vi "Kinect Led Options.vi"(4 "Clear":bool, 6 "Rec":bool, 8 "States":T2, 9 "Bye active":bool, 10 "Bye inactive":bool) -> (0 "Led Option":T1)   [LabVIEW 2015]
uses:
  TypeDefs Host/States.ctl
  Kinect Support/Controls/Led Control.ctl
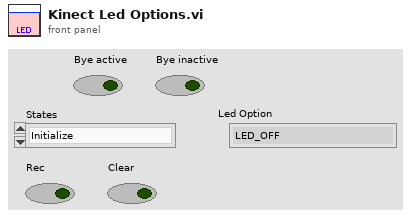
[diagram p1: front panel]
types:
  T1 = typedef "Led Control.ctl" = enum32{"LED_OFF", "LED_GREEN", "LED_RED", "LED_YELLOW", "LED_BLINK_GREEN", "LED_BLINK_GREEN2", "LED_BLINK_RED_YELLOW"}
  T2 = typedef "States.ctl" = enum16{"Initialize", "Calibrate", "Create", "Settings", "Shutdown"}
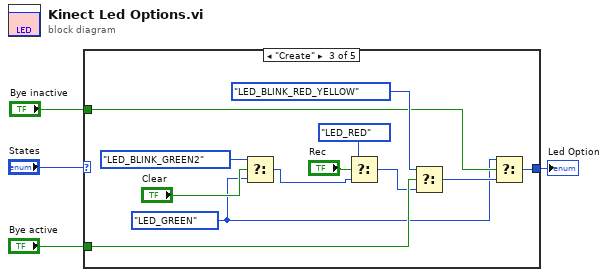
[diagram p0: block diagram]
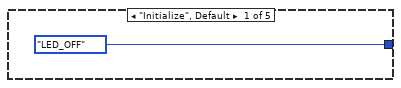
[diagram p2: hidden frame]
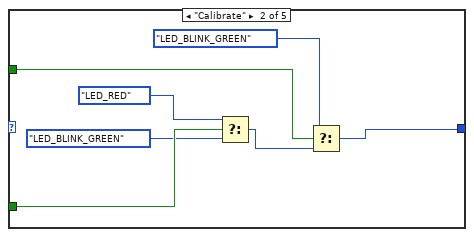
[diagram p3: hidden frame]
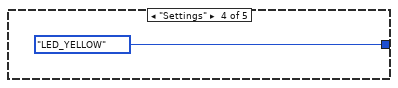
[diagram p4: hidden frame]
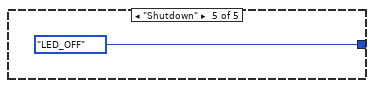
[diagram p5: hidden frame]
diagram:
  n1 = case shown="\"Create\"" "States" {
    tunnel: [Led_Control."LED_OFF" ("Led Option") w9 w16 Led_Control."LED_YELLOW" ("Led Option") Led_Control."LED_OFF" ("Led Option")] -> w3
    tunnel: "Bye active" -> [_ w12 w19 _ _]
    tunnel: "Bye inactive" -> [_ w8 w15 _ _]
    frame "Initialize", Default {
    }
    frame "Calibrate" {
      n2 = Select(t=Led_Control."LED_RED" ("Led Option"), s=w12, f=Led_Control."LED_BLINK_GREEN" ("Led Option")) -> (s? t:f=w7:T1)
      n3 = Select(t=Led_Control."LED_BLINK_GREEN", s=w8, f=w7) -> (s? t:f=w9:T1)
    }
    frame "Create" {
      w13 = Led_Control."LED_GREEN" ("Led Option")
      n4 = Select(t=Led_Control."LED_BLINK_GREEN2", s="Clear", f=w13) -> (s? t:f=w22:T1)
      n5 = Select(t=Led_Control."LED_RED" ("Led Option"), s="Rec", f=w22) -> (s? t:f=w18:T1)
      n6 = Select(t=Led_Control."LED_BLINK_RED_YELLOW" ("Led Option"), s=w19, f=w18) -> (s? t:f=w14:T1)
      n7 = Select(t=w13, s=w15, f=w14) -> (s? t:f=w16:T1)
    }
    frame "Settings" {
    }
    frame "Shutdown" {
    }
  }
  "Led Option" <- w3
